vi "FRCts20_Backend_Stats_Reform_GlobalSW.vi"(8 "Error In":errorcluster, 11 "data":cluster{"SWType":string, "Number":dbl}[](array[cluster])) -> (0 "Error Out":errorcluster, 3 "Software Usage Pie":T1)   [LabVIEW 2014, in "FRCts20_Backend_Engine.lvlib"]
uses:
  FRCts20_Backend_Engine.lvlib
  FRCts20_Backend_API/FRCts20_Backend_API_Stats.ctl
  ESP Engine/source/VI Source/TypeDefs/FRCts20_EspEngine_RequestPerHour_Line.ctl
  ESP Engine/source/VI Source/TypeDefs/FRCts20_EspEngine_SwUsage_Pie.ctl
  ESP Engine/source/VI Source/TypeDefs/FRCts20_EspEngine_AdvancedComponents_Bar.ctl
  ESP Engine/source/VI Source/FRCts20_EspEngine.lvlib
  FRCts20_Backend_API/FRCts20_Backend_API.lvlib
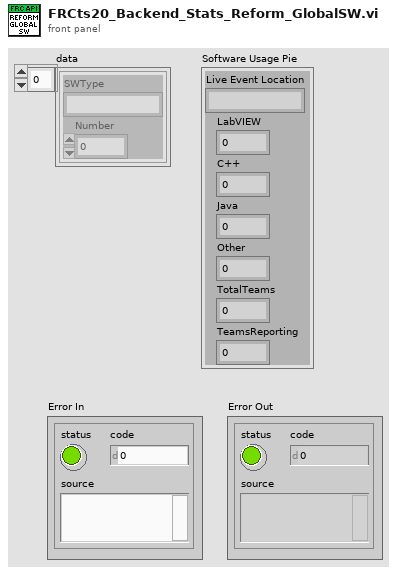
[diagram p1: front panel]
types:
  T1 = cluster{"Live Event Location":string, "LabVIEW":dbl, "C++":dbl, "Java":dbl, "Other":dbl, "TotalTeams":i32, "TeamsReporting":i32}
  T2 = typedef "FRCts20_Backend_API.lvlib/FRCts20_Backend_API_Stats.ctl" = cluster{"RequestsPerHour":T3, "SW Usage Pies":T4, "Advanced Components":T5, "APIReturn":string}
  T3 = typedef "FRCts20_EspEngine.lvlib/FRCts20_EspEngine_RequestPerHour_Line.ctl" = cluster{"StartDate":cluster{"Year":i32, "Month":i32, "Day":i32}, "Events":cluster{"Location":string, "Requests":i32[]}[]}
  T4 = typedef "FRCts20_EspEngine.lvlib/FRCts20_EspEngine_SwUsage_Pie.ctl" = cluster{"Live Event Location":string, "LabVIEW":dbl, "C++":dbl, "Java":dbl, "Other":dbl, "TotalTeams":i32, "TeamsReporting":i32}[]
  T5 = typedef "FRCts20_EspEngine.lvlib/FRCts20_EspEngine_AdvancedComponents_Bar.ctl" = cluster{"CAN":i32, "Vision":i32, "Kinect":i32}
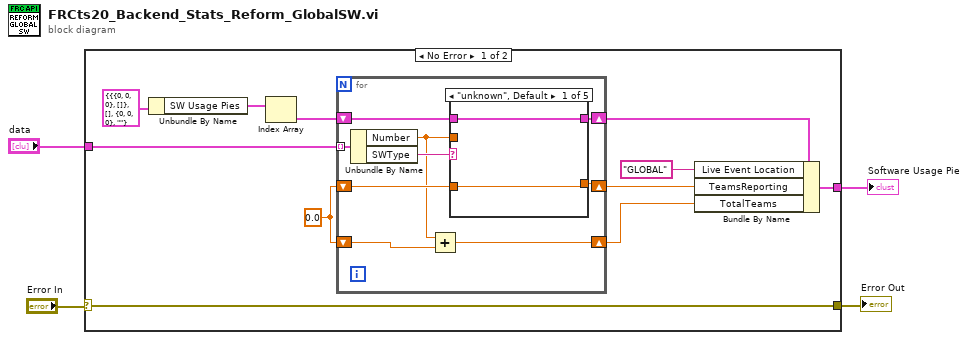
[diagram p0: block diagram]
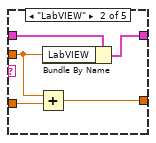
[diagram p2: hidden frame]
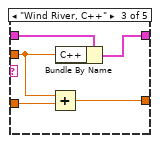
[diagram p3: hidden frame]
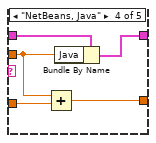
[diagram p4: hidden frame]
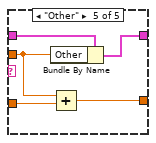
[diagram p5: hidden frame]
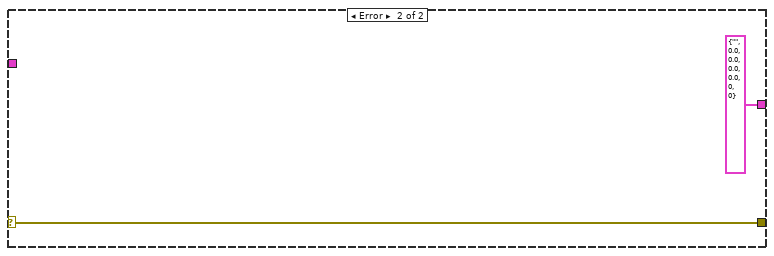
[diagram p6: hidden frame]
diagram:
  n1 = case shown="No Error" "Error In" {
    selector: "Error In" -> [w5 w48]
    tunnel: [w15 T1 {"Live Event Location"="", "LabVIEW"=0.0, "C++"=0.0, "Java"=0.0, "Other"=0.0, "TotalTeams"=0, "TeamsReporting"=0} ("Software Usage Pie")] -> w4
    tunnel: "data" -> [w6 _]
    tunnel: [w5 w48] -> w1
    frame No Error {
      w9 = 0.0 ("Number")
      n2 = Unbundle By Name(T2 {"RequestsPerHour"={"StartDate"={"Year"=0, "Month"=0, "Day"=0}, "Events"=[]}, "SW Usage Pies"=[], "Advanced Components"={"CAN"=0, "Vision"=0, "Kinect"=0}, "APIReturn"=""} ("Statistics")) -> ("SW Usage Pies"=w7:T4)
      n3 = Index Array(array=w7) -> (element=w8:T1)  [unwired: 1 in]
      n4 = for {
        tunnel: w6 -> [w24] mode=indexing
        shift-right: [w21] -> w10
        shift-left: w8 -> [w22]
        shift-right: [w18] -> w12
        shift-left: w9 -> [w20]
        shift-right: [w16] -> w11
        shift-left: w9 -> [w19]
        n5 = Unbundle By Name(w24) -> ("Number"=w17:dbl, "SWType"=w23:string)
        n6 = Add(x=w17, y=w20) -> (x+y=w18:dbl)
        n7 = case shown="\"unknown\", Default" w23 {
          tunnel: w22 -> [w26 w31 w36 w41 w46]
          tunnel: [w26 w30 w35 w40 w45] -> w21
          tunnel: w17 -> [_ w28 w33 w38 w43]
          tunnel: w19 -> [w25 w29 w34 w39 w44]
          tunnel: [w25 w27 w32 w37 w42] -> w16
          frame "unknown", Default {
          }
          frame "LabVIEW" {
            n8 = Add(x=w28, y=w29) -> (x+y=w27:dbl)
            n9 = Bundle By Name(cluster=w31, "LabVIEW"=w28) -> (w30:T1)
          }
          frame "Wind River, C++" {
            n10 = Add(x=w33, y=w34) -> (x+y=w32:dbl)
            n11 = Bundle By Name(cluster=w36, "C++"=w33) -> (w35:T1)
          }
          frame "NetBeans, Java" {
            n12 = Add(x=w38, y=w39) -> (x+y=w37:dbl)
            n13 = Bundle By Name(cluster=w41, "Java"=w38) -> (w40:T1)
          }
          frame "Other" {
            n14 = Bundle By Name(cluster=w46, "Other"=w43) -> (w45:T1)
            n15 = Add(x=w43, y=w44) -> (x+y=w42:dbl)
          }
        }
      }
      n16 = Bundle By Name(cluster=w10, "Live Event Location"="GLOBAL", "TeamsReporting"=w11, "TotalTeams"=w12) -> (w15:T1)
    }
    frame Error {
    }
  }
  "Software Usage Pie" <- w4
  "Error Out" <- w1
